vi "fxp_mult_fpga.vi"() -> ()   [LabVIEW 2009]
panel:
  in  "Accumulator Increment":u32
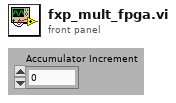
[diagram p1: front panel]
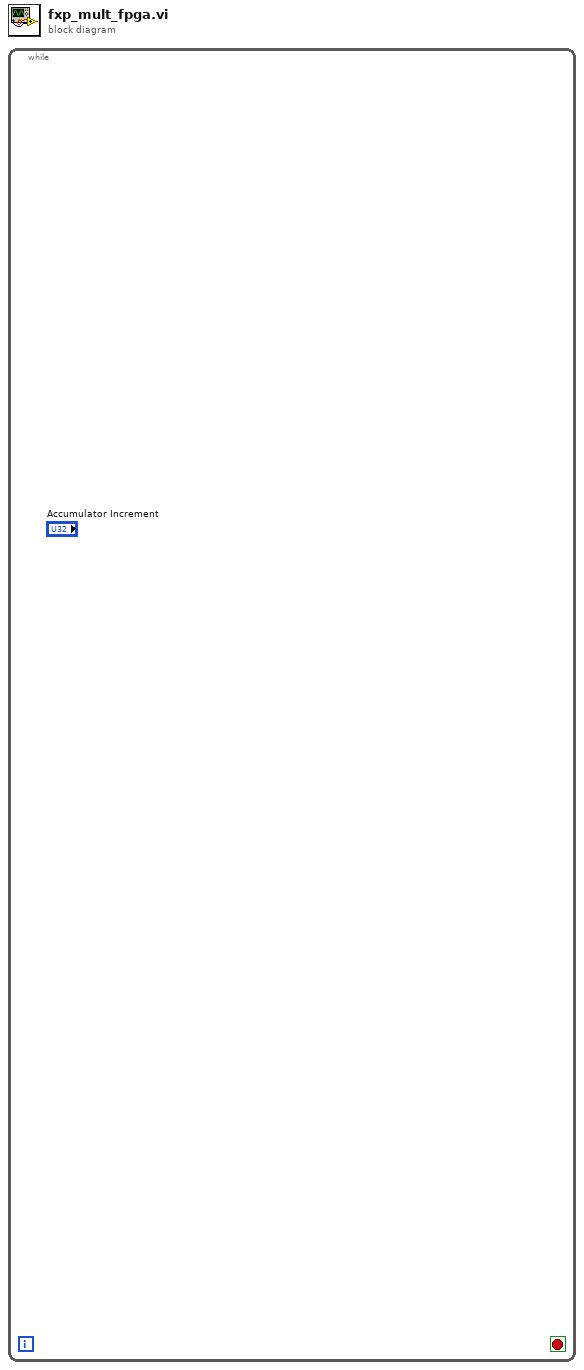
[diagram p0: block diagram]
diagram:
  n1 = while {
    stop <- _ stop-if-true
  }
